vi "Configure Multi Eval Meas Limit OBW.vi"(6 "OBW Limit (0.0)":dbl format="%^.3e", 7 "OBW Limit Enabled (Off)":bool, 8 "error in (no error)":errorcluster, 9 "Bandwidth (50 MHz)":T1 items=["50 MHz", "100 MHz", "200 MHz", "400 MHz"], 10 "Instance (1)":T2=1, 11 "VISA resource name":refnum<visa-resource-name>) -> (0 "error out":errorcluster, 3 "VISA resource name out":refnum<visa-resource-name>)   [LabVIEW 2015, in "Rohde&Schwarz CMXP NR FR2 Measurement.lvlib"]
doc: "Defines an upper limit for the occupied bandwidth, depending on the channel bandwidth.\n\nAttributes:\nRSCMXPNRFR2M_ATTR_MULTI_EVAL_MEASUREMENT_LIMIT_OBW\nRSCMXPNRFR2M_ATTR_MULTI_EVAL_MEASUREMENT_LIMIT_OBW_ENABLED\n\nRemote-control command:\nCONFigure:NRMMw:MEAS<i>:MEValuation:LIMit:SEMask:OBWLimit:CBANdwidth<bw>"
uses:
  <instrlib>/Rohde&Schwarz CMXP NR FR2 Measurement/Rohde&Schwarz CMXP NR FR2 Measurement.lvlib
  <instrlib>/Rohde&Schwarz CMXP NR FR2 Measurement/Private/_Instance.ctl
  <instrlib>/Rohde&Schwarz CMXP NR FR2 Measurement/Private/_Bandwidth.ctl
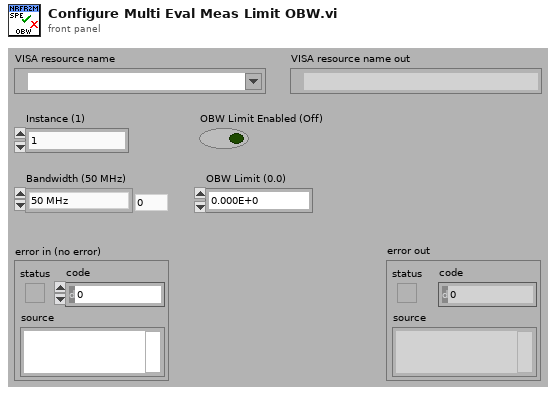
[diagram p1: front panel]
types:
  T1 = typedef "Rohde&Schwarz CMXP NR FR2 Measurement.lvlib/_Bandwidth.ctl" = i32
  T2 = typedef "Rohde&Schwarz CMXP NR FR2 Measurement.lvlib/_Instance.ctl" = i32
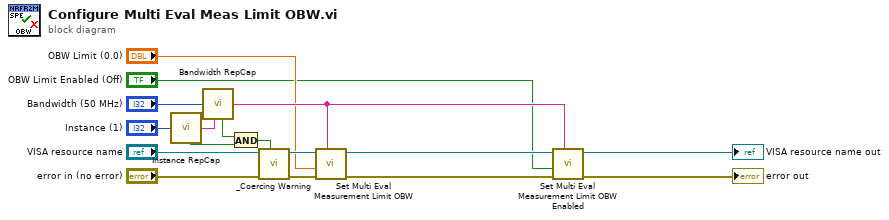
[diagram p0: block diagram]
diagram:
  n1 = call <instrlib>:"Instance RepCap.vi"("Instance In"="Instance (1)") -> ("In Range?"=w15:bool, "RepCap Identifier Out"=w3:string)  [unwired: 1 in]
  n2 = call <instrlib>:"Bandwidth RepCap.vi"("Bandwidth In"="Bandwidth (50 MHz)", "RepCap String In (\"\")"=w3) -> ("In Range?"=w14:bool, "RepCap Identifier Out"=w9:string)
  n3 = And(x=w14, y=w15) -> (x .and. y?=w13:bool)
  n4 = call <instrlib>:"_Coercing Warning.vi"("In Range?"=w13, "error in (no error)"="error in (no error)", "VISA resource name"="VISA resource name") -> ("error out"=w10:errorcluster, "VISA resource name out"=w11:refnum<visa-resource-name>)  [unwired: 7 in]
  n5 = call "Set Multi Eval Measurement Limit OBW"("Repeated Capabilities"=w9, "error in (no error)"=w10, "Multi Eval Measurement Limit OBW (0.0)"="OBW Limit (0.0)", "instrument handle"=w11) -> ("error out"=w7:errorcluster, "instrument handle out"=w8:refnum<visa-resource-name>)  [unwired: 6 in]
  n6 = call "Set Multi Eval Measurement Limit OBW Enabled"("Repeated Capabilities"=w9, "error in (no error)"=w7, "Multi Eval Measurement Limit OBW Enabled (OFF)"="OBW Limit Enabled (Off)", "instrument handle"=w8) -> ("error out"=→"error out":errorcluster, "instrument handle out"=→"VISA resource name out":refnum<visa-resource-name>)  [unwired: 6 in]
